vi "systemErrorClusterReplacement.vi"   [LabVIEW 2017, in "vi_tools.lvlib"]
doc: "From the front panel or block diagram window of a VI or a VI is selected on the File Dialog, select <b>Tools»System Error Cluster Replacement</b> to replace all Error clusters (in and out) on the VI front panel with System Error cluster.\n\nFrom the a project or lvlib explorer window or a folder is selected on the File Dialog, select <b>Tools»System Error Cluster Replacement</b> to replace all Error clusters (in and out) on all VI front panels with System Error cluster within the project or lvlib or user selected folder on disk."
uses:
  vi_tools.lvlib
types:
  T1 = enum32{"Invalid", "Standard", "Closed", "Hidden", "Minimized", "Maximized"}
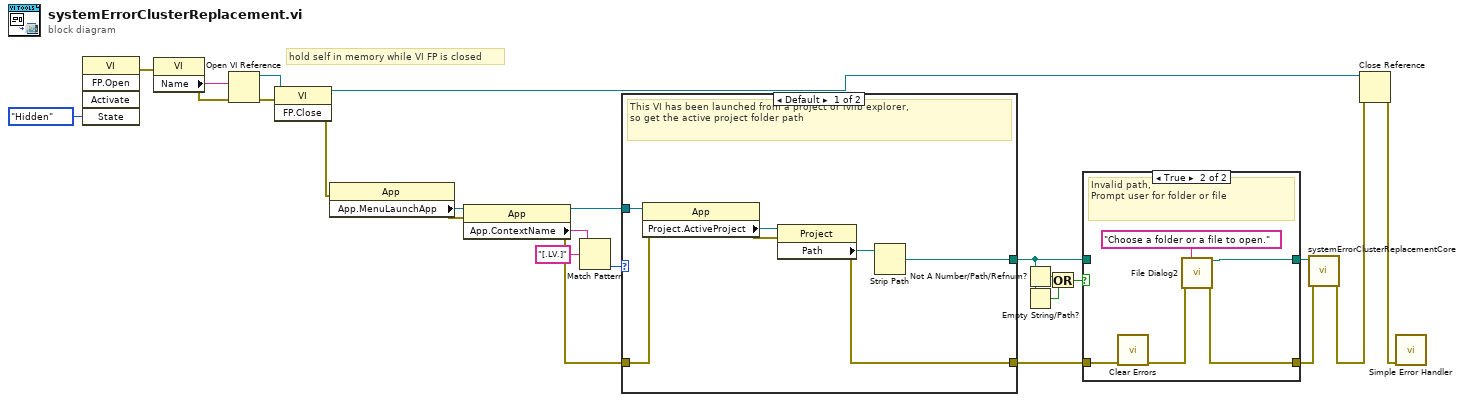
[diagram p0: block diagram]
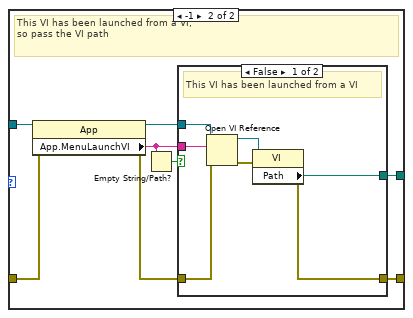
[diagram p3: hidden frame]
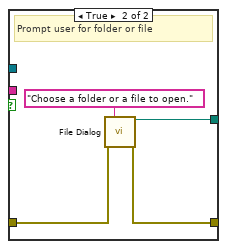
[diagram p4: hidden frame]
diagram:
  # "hold self in memory while VI FP is closed"
  n1 = invoke class="VI" method="FP.Open"("State"=T1."Hidden") -> (error out=w13:errorcluster)  [unwired: 4 in, 4 out]
  n2 = property class="VI"(error in=w13) -> (error out=w15:errorcluster, "Name"=w17:string)  [unwired: 1 in, 1 out]
  n3 = Open VI Reference(vi path=w17, error in (no error)=w15) -> (vi reference=w4:refnum<vi>, error out=w1:errorcluster)  [unwired: 4 in]
  n4 = invoke class="VI" method="FP.Close"(reference=w4, error in=w1) -> (reference out=w3:refnum<vi>, error out=w2:errorcluster)  [unwired: 1 in, 1 out]
  n5 = property class="App"(error in=w2) -> (error out=w21:errorcluster, "App.MenuLaunchApp"=w24:refnum<vi>)  [unwired: 1 in, 1 out]
  n6 = property class="App"(reference=w24, error in=w21) -> (reference out=w19:refnum<vi>, error out=w18:errorcluster, "App.ContextName"=w23:string)
  n7 = Match Pattern(string=w23, regular expression="[.LV.]") -> (offset past match=w20:i32)  [unwired: 1 in, 3 out]
  n8 = case shown="Default" w20 {
    tunnel: w19 -> [w29 w39]
    tunnel: w18 -> [w28 w36]
    tunnel: [w27 w32] -> w10
    tunnel: [w25 w33] -> w8
    frame Default {
      # "This VI has been launched from a project or lvlib explorer, \nso get the active project folder path"
      n9 = property class="App"(reference=w29, error in=w28) -> (error out=w30:errorcluster, "Project.ActiveProject"=w31:refnum<vi>)  [unwired: 1 out]
      n10 = property class="Project"(reference=w31, error in=w30) -> (error out=w27:errorcluster, "Path"=w26:path)  [unwired: 1 out]
      n11 = Strip Path(path=w26) -> (stripped path=w25:path)  [unwired: 1 out]
    }
    frame -1 {
      # "This VI has been launched from a VI,\nso pass the VI path"
      n12 = property class="App"(reference=w39, error in=w36) -> (reference out=w34:refnum<vi>, error out=w35:errorcluster, "App.MenuLaunchVI"=w37:string)
      n13 = Empty String/Path?(string/path=w37) -> (empty?=w38:bool)
      n14 = case shown="False" w38 {
        tunnel: w37 -> [w46 _]
        tunnel: w35 -> [w44 w48]
        tunnel: [w41 w47] -> w32
        tunnel: w34 -> [w45 _]
        tunnel: [w40 w50] -> w33
        frame False {
          # "This VI has been launched from a VI"
          n15 = Open VI Reference(application reference (local)=w45, vi path=w46, error in (no error)=w44) -> (vi reference=w42:refnum<vi>, error out=w43:errorcluster)  [unwired: 3 in]
          n16 = property class="VI"(reference=w42, error in=w43) -> (error out=w41:errorcluster, "Path"=w40:path)  [unwired: 1 out]
        }
        frame True {
          # "Prompt user for folder or file"
          n17 = call "File Dialog"("prompt"="Choose a folder or a file to open.", "error in"=w48) -> ("selected path"=w50:path, "error out"=w47:errorcluster)  [unwired: 10 in, 2 out]
        }
      }
    }
  }
  n18 = Not A Number/Path/Refnum?(number/path/refnum=w8) -> (NaN/Path/Refnum?=w11:bool)
  n19 = Empty String/Path?(string/path=w8) -> (empty?=w6:bool)
  n20 = Or(x=w11, y=w6) -> (x .or. y?=w7:bool)
  n21 = case shown="True" w7 {
    tunnel: [w52 w56] -> w12
    tunnel: w8 -> [w52 _]
    tunnel: w10 -> [w51 w54]
    tunnel: [w51 w55] -> w9
    frame False {
      # "Valid path"
    }
    frame True {
      # "Invalid path,\nPrompt user for folder or file"
      n22 = call <vilib>:"Clear Errors.vi"("error in (no error)"=w54) -> ("error out"=w53:errorcluster)  [unwired: 5 in, 1 out]
      n23 = call "File Dialog2"("prompt"="Choose a folder or a file to open.", "error in"=w53) -> ("selected path"=w56:path, "error out"=w55:errorcluster)  [unwired: 10 in, 2 out]
    }
  }
  n24 = call "systemErrorClusterReplacementCore.vi"("error in (no error)"=w9, "Folder Path"=w12) -> ("error out"=w14:errorcluster)  [unwired: 9 in]
  n25 = Close Reference(reference=w3, error in (no error)=w14) -> (error out=w5:errorcluster)
  n26 = call <vilib>:"Simple Error Handler.vi"("error in (no error)"=w5) -> ()  [unwired: 4 in, 5 out]
